vi "Initialise Intensity Chart.vi"(8 "error in (no error)":errorcluster) -> (0 "error out":errorcluster, 3 "Array":dbl[][](array[numeric]))   [LabVIEW 2017]
doc: "Initialises the intensity chart history array."
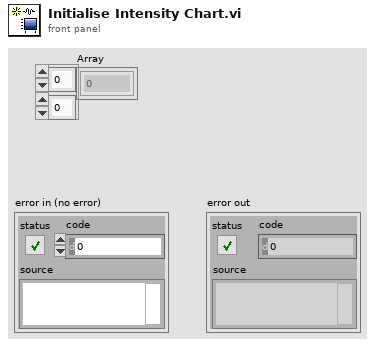
[diagram p1: front panel]
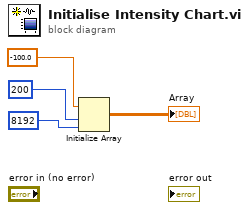
[diagram p0: block diagram]
diagram:
  n1 = Initialize Array(-100.0, 200 ("dimension size"), 8192 ("dimension size")) -> (→"Array":dbl[][])
